vi "Query Frequency Reference Status.vi"(0 "VISA resource name":refnum<visa-resource-name>, 11 "error in (no error)":errorcluster) -> (4 "VISA resource name out":refnum<visa-resource-name>, 6 "Signal Source":i32(ring) items=["INT", "INTU", "EXT", "EXTU"], 8 "Frequency Reference Status":i32, 15 "error out":errorcluster)   [LabVIEW 2020, in "Anritsu Signal Analyzer Series.lvlib"]
doc: "Queries the reference status."
uses:
  Anritsu Signal Analyzer Series.lvlib
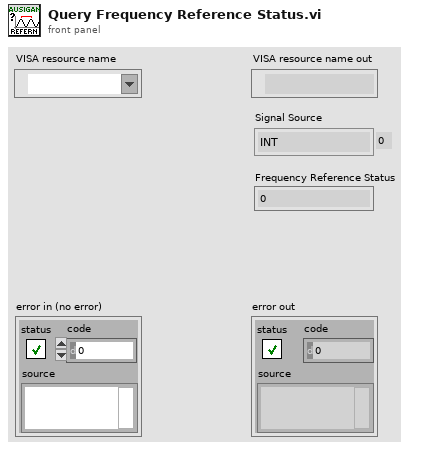
[diagram p1: front panel]
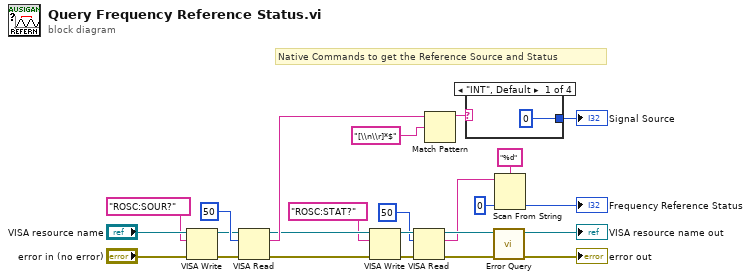
[diagram p0: block diagram]
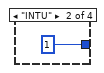
[diagram p2: hidden frame]
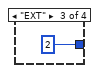
[diagram p3: hidden frame]
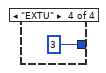
[diagram p4: hidden frame]
diagram:
  # "Native Commands to get the Reference Source and Status"
  n1 = VISA Write(VISA resource name="VISA resource name", write buffer="ROSC:SOUR?", error in (no error)="error in (no error)") -> (VISA resource name out=w14:refnum<visa-resource-name>, error out=w13:errorcluster)  [unwired: 1 out]
  n2 = VISA Read(VISA resource name=w14, byte count=u32 50 ("byte count (0)"), error in (no error)=w13) -> (VISA resource name out=w9:refnum<visa-resource-name>, read buffer=w17:string, error out=w8:errorcluster)  [unwired: 1 out]
  n3 = VISA Write(VISA resource name=w9, write buffer="ROSC:STAT?", error in (no error)=w8) -> (VISA resource name out=w12:refnum<visa-resource-name>, error out=w10:errorcluster)  [unwired: 1 out]
  n4 = VISA Read(VISA resource name=w12, byte count=u32 50 ("byte count (0)"), error in (no error)=w10) -> (VISA resource name out=w7:refnum<visa-resource-name>, read buffer=w3:string, error out=w6:errorcluster)  [unwired: 1 out]
  n5 = Match Pattern(string=w17, regular expression="[\\n\\r]*$") -> (before substring=w18:string)  [unwired: 1 in, 3 out]
  n6 = case shown="\"INT\", Default" w18 {
    tunnel: [0 ("source") 1 ("source") 2 ("source") 3 ("source")] -> w21
    frame "INT", Default {
    }
    frame "INTU" {
    }
    frame "EXT" {
    }
    frame "EXTU" {
    }
  }
  "Signal Source" <- w21
  n7 = call "Error Query.vi"("error in (no error)"=w6, "VISA resource name"=w7) -> ("error out"=→"error out":errorcluster, "VISA resource name out"=→"VISA resource name out":refnum<visa-resource-name>)  [unwired: 6 in, 2 out]
  n8 = Scan From String(format string="%d" ("Format String"), input string=w3, default 1=0 ("_Default")) -> (output 1=→"Frequency Reference Status":i32)  [unwired: 2 in, 3 out]
